vi "GPS Position.vi"() -> ()   [LabVIEW 2016]
panel:
  in  "Lat Long":string
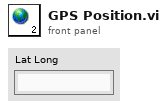
[diagram p1: front panel]
diagram:
